vi "Enable Disable.vi"() -> ()   [LabVIEW 2011, in "LVH-Adept.lvlib"]
uses:
  <vilib>/LabVIEW Hacker/Adept/LVH-Adept.lvlib
  <vilib>/LabVIEW Hacker/Adept/Private/DMGR/DMGR.lvlib
  <vilib>/LabVIEW Hacker/Adept/Private/DEPP/DEPP.lvlib
panel:
  out "Error Out":errorcluster
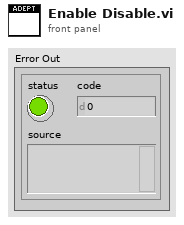
[diagram p1: front panel]
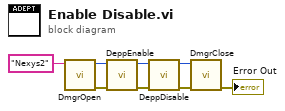
[diagram p0: block diagram]
diagram:
  n1 = call <vilib>:"DmgrOpen.vi"("Device Name"="Nexys2") -> ("Error Out"=w8:errorcluster, "Device Handle"=w3:u32)  [unwired: 9 in]
  n2 = call <vilib>:"DeppEnable.vi"("Error In"=w8, "Device Handle"=w3) -> ("Error Out"=w7:errorcluster, "Device Handle"=w4:u32)  [unwired: 8 in]
  n3 = call <vilib>:"DeppDisable.vi"("Error In"=w7, "Device Handle"=w4) -> ("Error Out"=w6:errorcluster, "Device Handle"=w5:u32)  [unwired: 8 in]
  n4 = call <vilib>:"DmgrClose.vi"("Error In"=w6, "hif"=w5) -> ("Error Out"=→"Error Out":errorcluster)  [unwired: 9 in]
